vi "GeoFonu_v1.2.vi"() -> ()   [LabVIEW 2014]
uses:
  <vilib>/Instr/_visa.llb/VISA Set IO Buffer Mask.ctl
  <vilib>/Instr/_visa.llb/VISA Flush IO Buffer Mask.ctl
  <vilib>/Instr/_visa.llb/VISA Configure Serial Port (Instr).vi
panel:
  in  "milliseconds to wait":u32=500
  in  "stop":bool
  in  "VISA resource name":refnum<visa-resource-name>
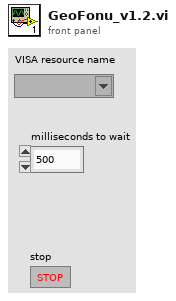
[diagram p1: front panel]
types:
  T1 = typedef "VISA Set IO Buffer Mask.ctl" = u16
  T2 = typedef "VISA Flush IO Buffer Mask.ctl" = u16
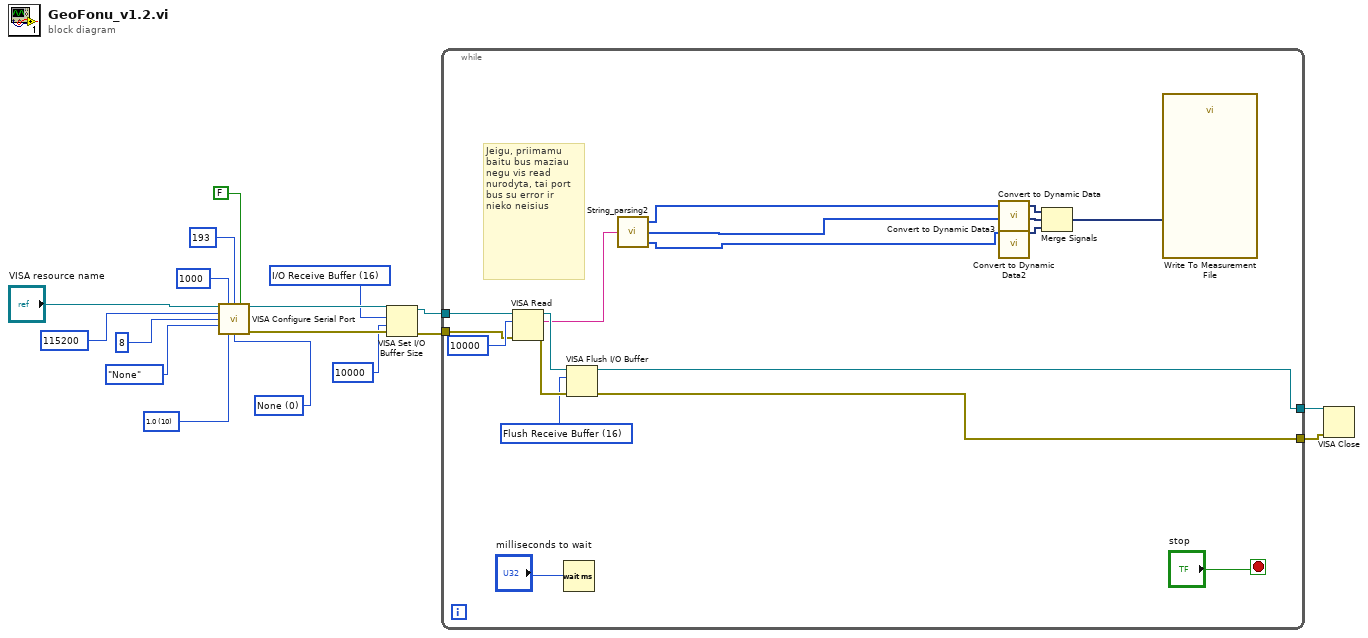
[diagram p0: block diagram]
diagram:
  w7 = T1 16 items=["I/O Receive Buffer"=16, "I/O Transmit Buffer"=32, "I/O Receive and Transmit Buffer"=48] ("Mask")
  w13 = u16 0 items=["None", "XON/XOFF", "RTS/CTS", "XON/XOFF & RTS/CTS", "DTR/DSR", "XON/XOFF & DTR/DSR"] ("flow control (0:none)")
  w14 = u16 10 items=["1.0"=10, "1.5"=15, "2.0"=20] ("stop bits (10: 1 bit)")
  n1 = call-poly "VISA Configure Serial Port"("VISA resource name"="VISA resource name", "timeout (10sec)"=u32 1000, "termination char\n(0xA = '\\n' = LF)"=u8 193 ("termination char\n(0xA = '\\n' = LF)"), "Enable Termination\nChar (T)"=FALSE ("Enable Termination\nChar (T)"), "baud rate (9600)"=u32 115200, "data bits (8)"=u16 8, "parity (0:none)"=enum16{"None", "Odd", "Even", "Mark", "Space"}."None", "stop bits (10: 1 bit)"=w14, "flow control (0:none)"=w13) -> ("VISA resource name out"=w9:refnum<visa-resource-name>, "error out"=w10:errorcluster)  [unwired: 5 in]
  n2 = VISA Set I/O Buffer Size(VISA resource name=w9, mask (16)=w7, size (4096)=u32 10000, error in (no error)=w10) -> (VISA resource name out=w3:refnum<visa-resource-name>, error out=w6:errorcluster)
  n3 = while {
    tunnel: w3 -> [w35]
    tunnel: w6 -> [w32]
    tunnel: [w26] -> w2
    tunnel: [w25] -> w1
    stop <- "stop" stop-if-true
    w29 = T2 16 items=["Flush Receive Buffer"=16, "Write Transmit Buffer to Device"=32, "Flush Receive Buffer (No I/O)"=64, "Flush Transmit Buffer"=128] ("Mask")
    # "Jeigu, priimamu baitu bus maziau negu vis read nurodyta, tai port bus su error ir nieko neisius"
    n4 = VISA Read(VISA resource name=w35, byte count=u32 10000, error in (no error)=w32) -> (VISA resource name out=w31:refnum<visa-resource-name>, read buffer=w27:string, error out=w30:errorcluster)  [unwired: 1 out]
    n5 = Wait (ms)(milliseconds to wait="milliseconds to wait") -> ()  [unwired: 1 out]
    n6 = VISA Flush I/O Buffer(VISA resource name=w31, mask (16)=w29, error in (no error)=w30) -> (VISA resource name out=w26:refnum<visa-resource-name>, error out=w25:errorcluster)
    n7 = call "String_parsing2.vi"("input string"=w27) -> ("V3"=w21:i32[], "V2"=w19:i32[], "V1"=w24:i32[])  [unwired: 2 in]
    n8 = call "Convert to Dynamic Data"("Array"=w24) -> ("Dynamic Data Type"=w23:dynamicdata)  [unwired: 3 in]
    n9 = call "Convert to Dynamic Data3"("Array"=w19) -> ("Dynamic Data Type"=w18:dynamicdata)  [unwired: 3 in]
    n10 = call "Convert to Dynamic Data2"("Array"=w21) -> ("Dynamic Data Type"=w20:dynamicdata)  [unwired: 3 in]
    n11 = Merge Signals(w23, w18, w20) -> (w22:dynamicdata)
    n12 = call "Write To Measurement File"("Signals"=w22) -> ()  [unwired: 16 in, 3 out]
  }
  n13 = VISA Close(VISA resource name=w2, error in (no error)=w1) -> ()  [unwired: 1 out]
